vi "Get Approver ID.vi"(11 "Submission in":refnum<class "Submission.lvclass">) -> (2 "Approver ID":i64, 3 "Submission out":refnum<class "Submission.lvclass">)   [LabVIEW 2020, in "Summer of LabVIEW.lvlib" / "Submission.lvclass"]
uses:
  Submission.lvclass
  Submission.lvclass/Submission.ctl
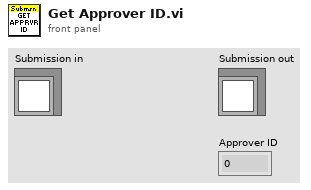
[diagram p1: front panel]
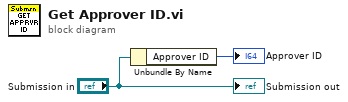
[diagram p0: block diagram]
diagram:
  n1 = Unbundle By Name("Submission in") -> ("Approver ID"=→"Approver ID":i64)
  "Submission out" <- "Submission in"
